vi "Verify Account.vi"(8 "error in (no error)":errorcluster, 10 "Account":string=",", 11 "Path Account File":path=path "C:/Users/jviquez/Desktop/CLD Simulator/CLD Preparation/Github-SourceTree/Excersise Solutions/Exam 3/Solution 1/ATM accounts.txt") -> (0 "error out":errorcluster, 3 "Account exist?":bool)   [LabVIEW 2020]
doc: "This VI verifies if the account information is valid."
uses:
  <vilib>/Utility/file.llb/Read Delimited Spreadsheet (string).vi
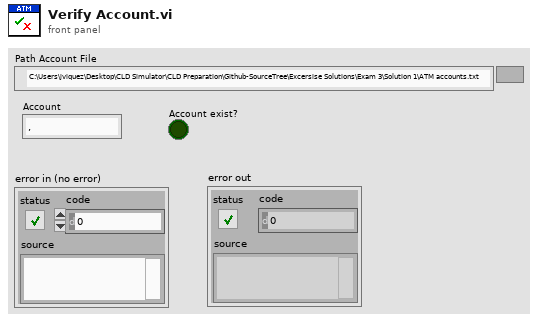
[diagram p1: front panel]
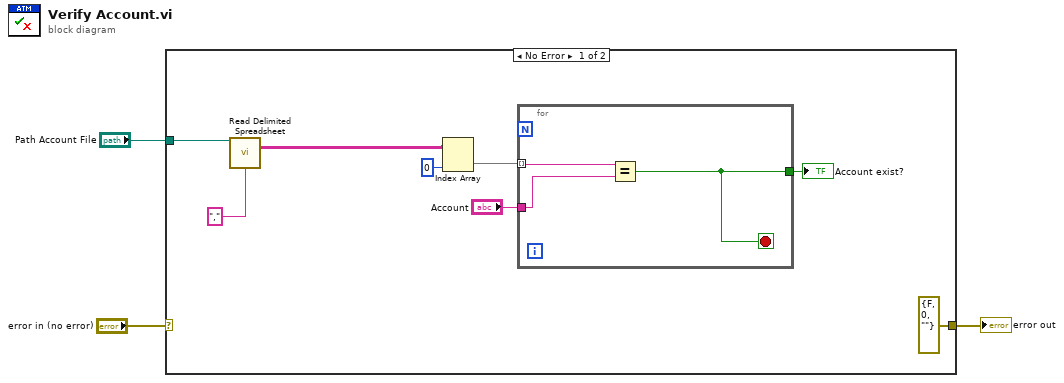
[diagram p0: block diagram]
diagram:
  n1 = case shown="No Error" "error in (no error)" {
    selector: "error in (no error)" -> [_ w15]
    tunnel: [errorcluster {"status"=FALSE, "code"=0, "source"=""} ("error IO") w15] -> w2
    tunnel: "Path Account File" -> [w11 _]
    frame No Error {
      n2 = call-poly <vilib>:"Read Delimited Spreadsheet.vi"("file path (dialog if empty)"=w11, "delimiter (\\t)"="," ("delimiter (\\t)")) -> ("all rows"=w9:string[][])  [unwired: 8 in, 5 out]
      n3 = Index Array(array=w9, index (col)=0 ("disabled index (col)")) -> (element=w7:string[])  [unwired: 1 in]
      n4 = for {
        tunnel: w7 -> [w14] mode=indexing
        tunnel: "Account" -> [w13]
        tunnel: [w12] -> w5
        stop <- w12 stop-if-true
        n5 = Equal?(x=w14, y=w13) -> (x = y?=w12:bool)
      }
      "Account exist?" <- w5
    }
    frame Error {
    }
  }
  "error out" <- w2
